vi "generate big random array.vi"(10 "dim 2":i32=100, 11 "dim 1":i32=100) -> (3 "Array":dbl[][](array[numeric]))   [LabVIEW 2018, in "LV2Julia_core.lvlib"]
uses:
  LV2Julia_core.lvlib
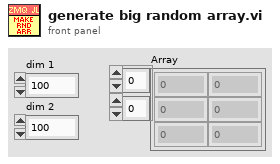
[diagram p1: front panel]
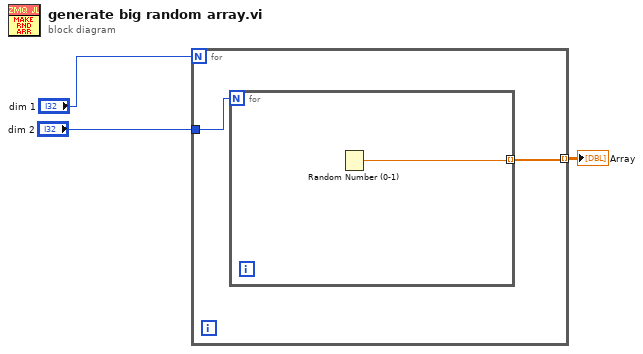
[diagram p0: block diagram]
diagram:
  n1 = for {
    N: "dim 1" -> [_]
    tunnel: "dim 2" -> [w5]
    tunnel: [w4] -> w1 mode=indexing
    n2 = for {
      N: w5 -> [_]
      tunnel: [w6] -> w4 mode=indexing
      n3 = Random Number (0-1)() -> (number: 0 to 1=w6:dbl)
    }
  }
  "Array" <- w1
